vi "Teleop.vi"(10 "Match Info":T1={"Autonomous Elapsed Seconds"=0.0, "TeleOp Elapsed Seconds"=0.0, "Disabled Elapsed Seconds"=0.0, "Visited Autonomous"=FALSE, "Visited TeleOp"=FALSE, "Visited Disabled"=FALSE, "Autonomous Settings"={"Autonomous Style"=enum."Independent", "VI Refnum"=refnum}}, 11 "Call Context":T2) -> ()   [LabVIEW 2025]
doc: "This VI is called for each enabled TeleOp packet received from the DS. It is typically used to read from joysticks and other inputs and update I/O or setpoints for timed control loops. It should complete and return within 20 milliseconds or risk missing DS packets."
uses:
  <vilib>/Rock Robotics/WPI/DriverStation/WPI_DriverStationDerivedRobotMode.ctl
  <vilib>/Rock Robotics/WPI/DriverStation/WPI_DriverStationMatch Info.ctl
  <vilib>/Rock Robotics/Network Tables/NT Read Numeric Array.vi
  Support Code/Globals.vi
  <vilib>/Rock Robotics/WPI/Utilities/WPI_GetSetVariantRefNum.vi
panel:
  out "Game Data Recieved?":bool
  out "value":dbl[](array[numeric])
  # "Avg Tag\nDist"
  # "Y"
  # "Z"
  # "Roll"
  # "Pitch"
  # "Yaw"
  # "Latency"
  # "X"
  # "Tag Cnt"
  # "Tag Span"
  # "tag ID"
  # "Driver Controls"
  # "Operator Controls"
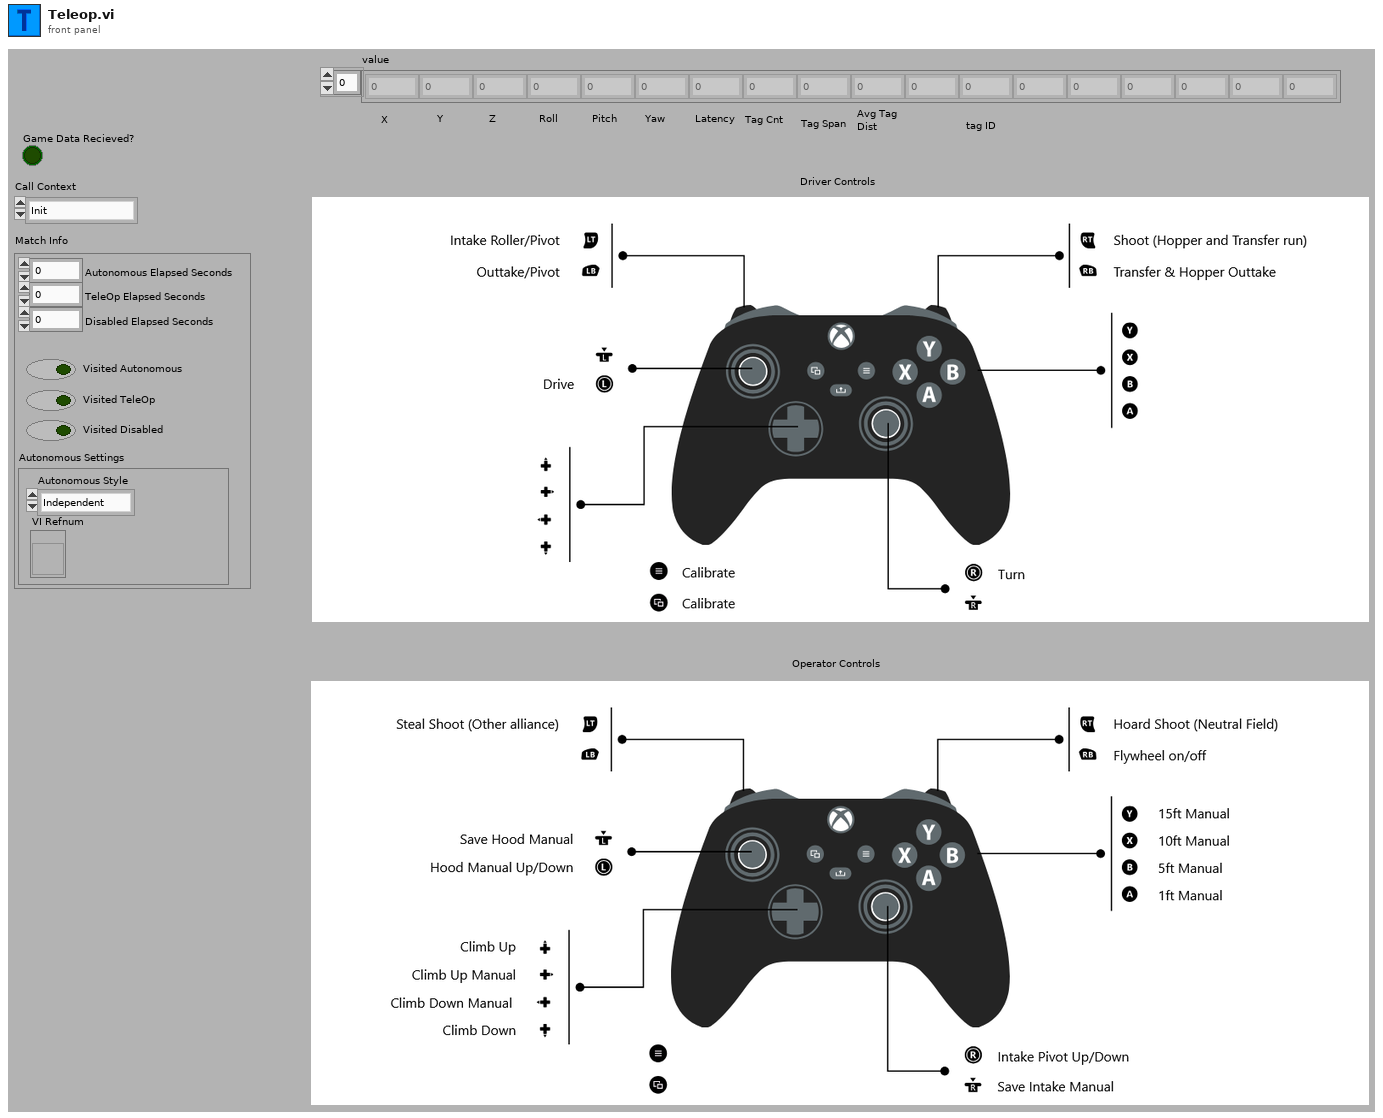
[diagram p1: front panel]
types:
  T1 = typedef "WPI_DriverStationMatch Info.ctl" = cluster{"Autonomous Elapsed Seconds":dbl, "TeleOp Elapsed Seconds":dbl, "Disabled Elapsed Seconds":dbl, "Visited Autonomous":bool, "Visited TeleOp":bool, "Visited Disabled":bool, "Autonomous Settings":cluster{"Autonomous Style":enum16{"Iterative", "Independent"}, "VI Refnum":refnum<vi>}}
  T2 = typedef "WPI_DriverStationDerivedRobotMode.ctl" = enum16{"Init", "Execute", "Stop"}
  T3 = typedef "Robot Velocities.ctl" = cluster{"X Velocity":dbl, "Y Velocity":dbl, "Rotational \nVelocity":dbl}
  T4 = typedef "WPI_JoystickDevRef.ctl" = cluster{"Device":T5}
  T5 = typedef "WPI_JoystickDeviceEnum.ctl" = enum16{"USB 0", "USB 1", "USB 2", "USB 3", "USB 4", "USB 5"}
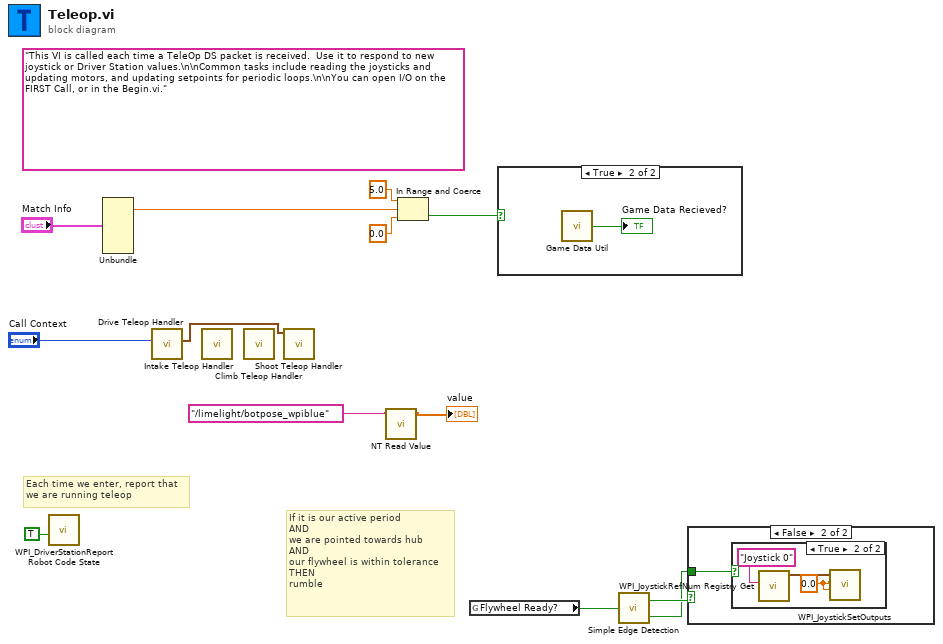
[diagram p0: block diagram]
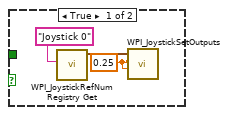
[diagram p2: hidden frame]
diagram:
  (unwired) "This VI is called each time a TeleOp DS packet is received.  Use it to respond to new joystick or Driver Station values.\n\nCommon tasks include reading the joysticks and updating motors, and updating setpoints for periodic loops.\n\nYou can open I/O on the FIRST Call, or in the Begin.vi."
  # "If it is our active period\nAND\nwe are pointed towards hub\nAND\nour flywheel is within tolerance\nTHEN\nrumble"
  # "Each time we enter, report that\nwe are running teleop"
  n1 = call <vilib>:"WPI_DriverStationReport Robot Code State.vi"("TeleOp"=TRUE ("Autonomous")) -> ()  [unwired: 10 in, 1 out]
  n2 = Unbundle("Match Info") -> ("TeleOp Elapsed Seconds"=w7:dbl)  [unwired: 6 out]
  n3 = call "Drive Teleop Handler.vi"("Call Context"="Call Context") -> ("Robot Velocities"=w9:T3)  [unwired: 10 in]
  n4 = call "Intake Teleop Handler.vi"() -> ()  [unwired: 12 in]
  n5 = call "Climb Teleop Handler.vi"() -> ()  [unwired: 12 in]
  n6 = call "Shoot Teleop Handler.vi"("Input Velocities"=w9) -> ()  [unwired: 11 in]
  n7 = call-poly <vilib>:"NT Read Value.vi"("name"="/limelight/botpose_wpiblue") -> ("value"=→"value":dbl[])  [unwired: 8 in, 2 out]
  n8 = In Range and Coerce(upper limit=5.0, x=w7, lower limit=0.0) -> (In Range?=w4:bool)  [unwired: 1 out]
  n9 = global read "Globals.vi" "Flywheel Ready?"() -> (w3:bool)
  n10 = case shown="True" w4 {
    frame False {
    }
    frame True {
      n11 = call "Game Data Util.vi"() -> ("Game Data Recieved?"=→"Game Data Recieved?":bool)  [unwired: 1 in]
    }
  }
  n12 = call "Simple Edge Detection.vi"("In"=w3) -> ("Rising Edge"=w2:bool, "Falling Edge"=w1:bool)
  n13 = case shown="False" w2 {
    tunnel: w1 -> [_ w18]
    frame True {
      w15 = sgl 0.25 ("Left Rumble")
      n14 = call <vilib>:"WPI_JoystickRefNum Registry Get.vi"("refnum name"="Joystick 0") -> ("JoystickDevRef"=w16:T4)  [unwired: 9 in, 1 out]
      n15 = call <vilib>:"WPI_JoystickSetOutputs.vi"("Right Rumble"=w15, "Left Rumble"=w15, "JoystickDevRef"=w16) -> ()  [unwired: 7 in, 2 out]
    }
    frame False {
      n16 = case shown="True" w18 {
        frame False {
        }
        frame True {
          w19 = sgl 0.0 ("Left Rumble")
          n17 = call <vilib>:"WPI_JoystickRefNum Registry Get.vi"("refnum name"="Joystick 0") -> ("JoystickDevRef"=w20:T4)  [unwired: 9 in, 1 out]
          n18 = call <vilib>:"WPI_JoystickSetOutputs.vi"("Right Rumble"=w19, "Left Rumble"=w19, "JoystickDevRef"=w20) -> ()  [unwired: 7 in, 2 out]
        }
      }
    }
  }
